vi "GEvt-Convert Filter Rules - Periodic Setting Only.vi"(11 "PeriodicMessageFilter":T1={"Enable"=TRUE, "Threshold(#/s)"=2.0, "CheckPeriod(s)"=1.0}) -> (3 "GlobalLogFilter":refnum<class "LogFilter.lvclass">)   [LabVIEW 2017, in "Communicable State Machine.lvlib"]
uses:
  Communicable State Machine.lvlib
  LogFilter/LogFilter.lvclass
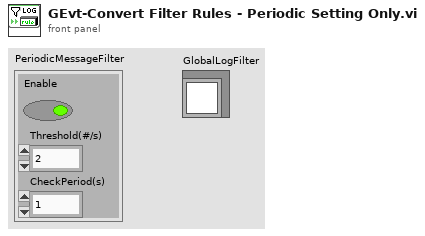
[diagram p1: front panel]
types:
  T1 = cluster{"Enable":bool, "Threshold(#/s)":dbl, "CheckPeriod(s)":dbl}
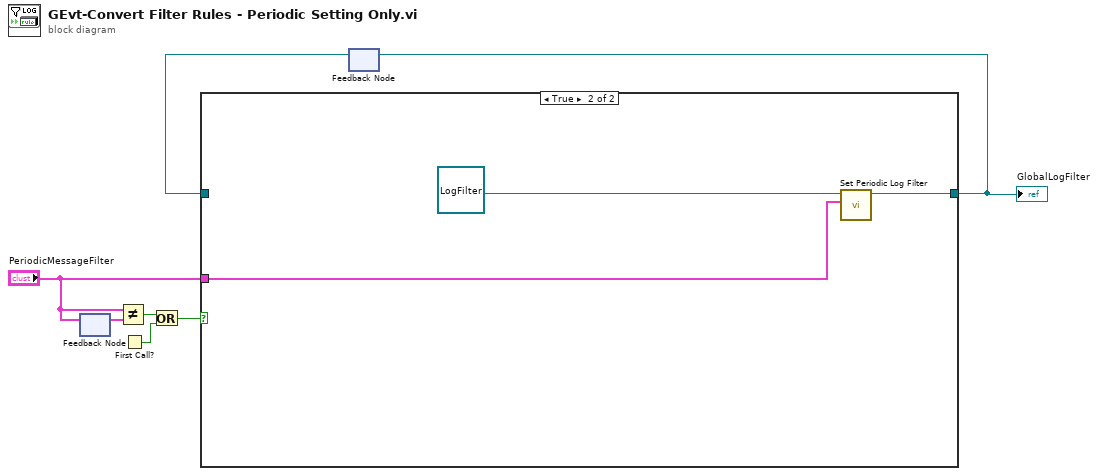
[diagram p0: block diagram]
diagram:
  n1 = feedback #1() -> (w2:T1)  [unwired: 1 in]
  n2 = feedback-in #1("PeriodicMessageFilter") -> ()
  n3 = Not Equal?(x="PeriodicMessageFilter", y=w2) -> (x != y?=w3:bool)
  n4 = First Call?() -> (First Call?: T/F=w4:bool)
  n5 = Or(x=w3, y=w4) -> (x .or. y?=w5:bool)
  n6 = feedback #2() -> (w7:refnum<class "LogFilter.lvclass">)  [unwired: 1 in]
  n7 = case shown="True" w5 {
    tunnel: [w8 w11] -> w6
    tunnel: "PeriodicMessageFilter" -> [_ w9]
    tunnel: w7 -> [w8 _]
    frame False {
    }
    frame True {
      n8 = call "Set Periodic Log Filter.vi"("PeriodicLogFilter"=w9, "GlobalLogFilter In"=refnum<class "LogFilter.lvclass"> refnum ("GlobalLogFilter.lvclass")) -> ("GlobalLogFilter Out"=w11:refnum<class "LogFilter.lvclass">)  [unwired: 9 in]
    }
  }
  "GlobalLogFilter" <- w6
  n9 = feedback-in #2(w6) -> ()
